vi "Test Sequencer.vi"() -> ()   [LabVIEW 2020]
uses:
  Sequencer.lvclass
  Test Steps/Types/Example Step/Example Step.lvclass
  Test Steps/Base Step/Base Step.lvclass
  Test Steps/Sequence/Sequence.lvclass
  Classes/Service/Service.lvclass
  Classes/Communications/Server/Base Server/Server.lvclass
  <vilib>/Utility/miscctls.llb/LVBoundsTypeDef.ctl
  C:/TestSystemServices/Total Fire Systems/Main/Tree/Classes/Service/Service.lvclass
  C:/TestSystemServices/Total Fire Systems/Main/Tree/Sequencer/Sequencer.lvclass
  C:/TestSystemServices/Total Fire Systems/Main/Tree/Test Steps/Base Step/Base Step.lvclass
  C:/TestSystemServices/Total Fire Systems/Main/Tree/Test Steps/Types/Example Step/Example Step.lvclass
panel:
  in  "Reset":bool
  in  "Start":bool
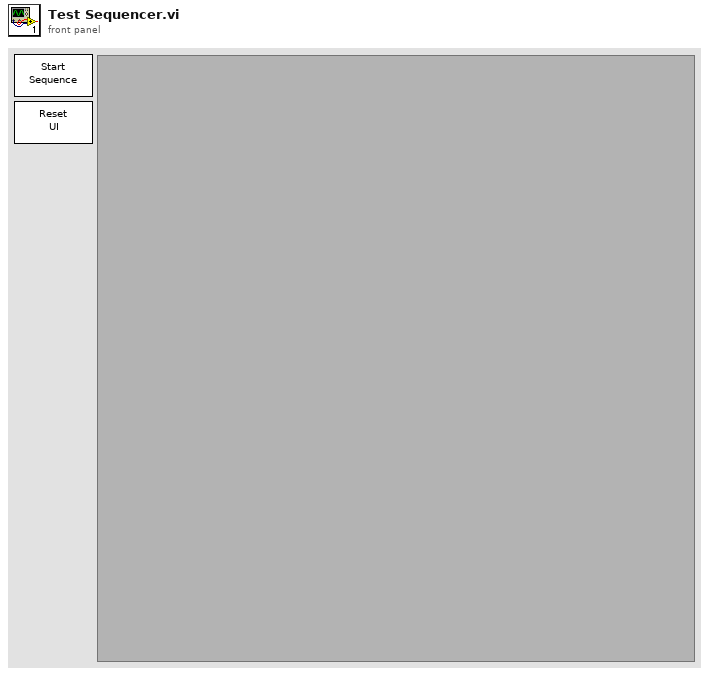
[diagram p1: front panel]
types:
  T1 = typedef "LVBoundsTypeDef.ctl" = cluster{"Width":u32, "Height":u32}
  T2 = typedef "LVPointTypeDef.ctl" = cluster{"Horizontal":i16, "Vertical":i16}
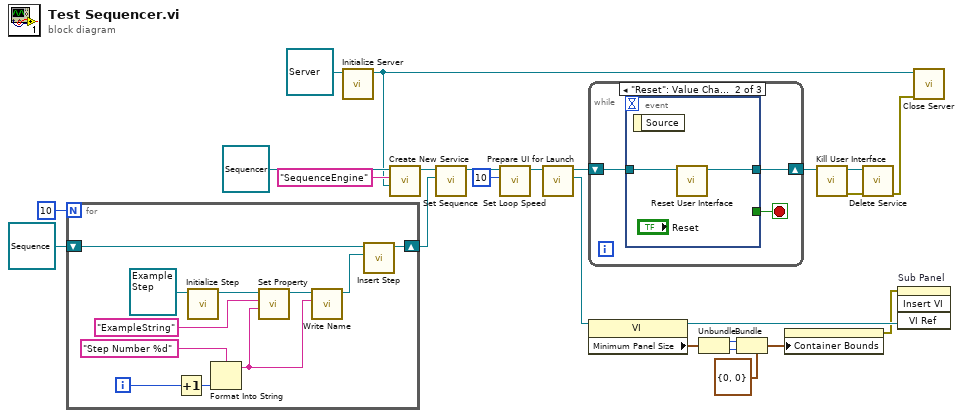
[diagram p0: block diagram]
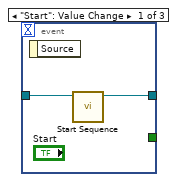
[diagram p2: hidden frame]
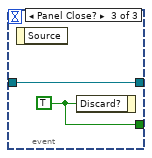
[diagram p3: hidden frame]
diagram:
  n1 = for {
    N: 10 -> [_]
    shift-right: [w30] -> w18
    shift-left: refnum<class "Sequence.lvclass"> refnum ("Sequence.lvclass") -> [w31]
    i -> [w34]
    n2 = Increment(x=w34) -> (x+1=w33:i32)
    n3 = call "Initialize Step.vi"("Base Step in"=refnum<class "Example Step.lvclass"> refnum ("Example Step.lvclass")) -> ("Base Step out"=w26:refnum<class "Example Step.lvclass">)  [unwired: 9 in, 1 out]
    n4 = Format Into String(format string="Step Number %d", w33) -> (resulting string=w27:string)  [unwired: 2 in, 1 out]
    n5 = call "Set Property.vi"("Data"=w27, "Key"="ExampleString", "Base Step in"=w26) -> ("Base Step out"=w29:refnum<class "Example Step.lvclass">)  [unwired: 7 in, 1 out]
    n6 = call-dynamic "Write Name.vi"("Name"=w27, "Base Step in"=w29) -> ("Base Step out"=w28:refnum<class "Example Step.lvclass">)  [unwired: 8 in, 1 out]
    n7 = call "Insert Step.vi"("Step"=w28, "Sequence in"=w31) -> ("Sequence out"=w30:refnum<class "Sequence.lvclass">)  [unwired: 8 in, 1 out]
  }
  n8 = call-dynamic "Initialize Server.vi"("Base Server in"=refnum<class "Server.lvclass"> refnum ("Server.lvclass")) -> ("Base Server out"=w17:refnum<class "Server.lvclass">)  [unwired: 9 in, 1 out]
  n9 = call "Create New Service.vi"("Server in"=w17, "Name"="SequenceEngine", "Service in"=refnum<class "Sequencer.lvclass"> refnum ("Sequencer.lvclass")) -> ("Service out"=w19:refnum<class "Sequencer.lvclass">)  [unwired: 7 in, 1 out]
  n10 = call "Set Sequence.vi"("Sequence"=w18, "Sequencer in"=w19) -> ("Service out"=w16:refnum<class "Sequencer.lvclass">)  [unwired: 8 in, 1 out]
  n11 = call "Set Loop Speed.vi"("Loop Speed"=10, "Service in"=w16) -> ("Service out"=w13:refnum<class "Sequencer.lvclass">)  [unwired: 8 in, 1 out]
  n12 = call "Prepare UI for Launch.vi"("Service in"=w13) -> ("UI Reference"=w8:refnum<vi>, "Service out"=w12:refnum<class "Sequencer.lvclass">)  [unwired: 8 in, 1 out]
  n13 = while {
    shift-right: [w37] -> w11
    shift-left: w12 -> [w38]
    stop <- w36 stop-if-true
    n14 = event shown="[1] \"Reset\": Value Change" {
      selector: _ -> [_ _ _]
      dyn-events: _ -> [_ _ _]
      timeout: _ -> [_ _ _]
      tunnel: w38 -> [w40 w42 w44]
      tunnel: [w39 w41 w44] -> w37
      tunnel: [_ _ w43] -> w36
      event "Start": Value Change {
        n15 = event-data() -> ()  [unwired: 1 in, 1 out]
        n16 = call "Start Sequence.vi"("Sequencer in"=w40) -> ("Sequencer out"=w39:refnum<class "Sequencer.lvclass">)  [unwired: 9 in, 1 out]
      }
      event "Reset": Value Change {
        n17 = event-data() -> ()  [unwired: 1 in, 1 out]
        n18 = call "Reset User Interface.vi"("Sequencer in"=w42) -> ("Sequencer out"=w41:refnum<class "Sequencer.lvclass">)  [unwired: 9 in, 1 out]
      }
      event Panel Close? {
        w43 = TRUE ("Discard?")
        n19 = event-data() -> ()  [unwired: 1 in, 1 out]
        n20 = event-data("Discard?"=w43) -> ()  [unwired: 1 in, 1 out]
      }
    }
  }
  n21 = property class="VI"(reference=w8) -> (reference out=w4:refnum<vi>, "Minimum Panel Size"=w7:T2)  [unwired: 1 in, 1 out]
  n22 = Unbundle(w7) -> ("Horizontal"=w2:i16, "Vertical"=w1:i16)
  n23 = Bundle(cluster=T1 {"Width"=0, "Height"=0} ("Container Bounds"), "Width"=w2, "Height"=w1) -> (w5:T1)
  n24 = property on="Sub Panel" class="SubPnl"("Container Bounds"=w5) -> (error out=w3:errorcluster)  [unwired: 2 in, 1 out]
  n25 = call "Kill User Interface.vi"("Service in"=w11) -> ("error out"=w9:errorcluster, "Service out"=w10:refnum<class "Sequencer.lvclass">)  [unwired: 9 in]
  n26 = call "Delete Service.vi"("error in (no error)"=w9, "Service in"=w10) -> ("error out"=w14:errorcluster)  [unwired: 9 in]
  n27 = invoke on="Sub Panel" class="SubPnl" method="Insert VI"(error in=w3, "VI Ref"=w4) -> ()  [unwired: 2 in, 4 out]
  n28 = call-dynamic "Close Server.vi"("error in (no error)"=w14, "Base Server in"=w17) -> ()  [unwired: 8 in, 2 out]
